vi "Boolean Array to Integer.vi"() -> ()   [LabVIEW 2010]
uses:
  <vilib>/DAQmx/write.llb/DAQmx Write (Digital 1D U8 1Chan NSamp).vi
panel:
  out "output array":u8[](array[numeric])
  out "unsigned 8bit integer":u8
  in  "Array":bool[](array[boolean])
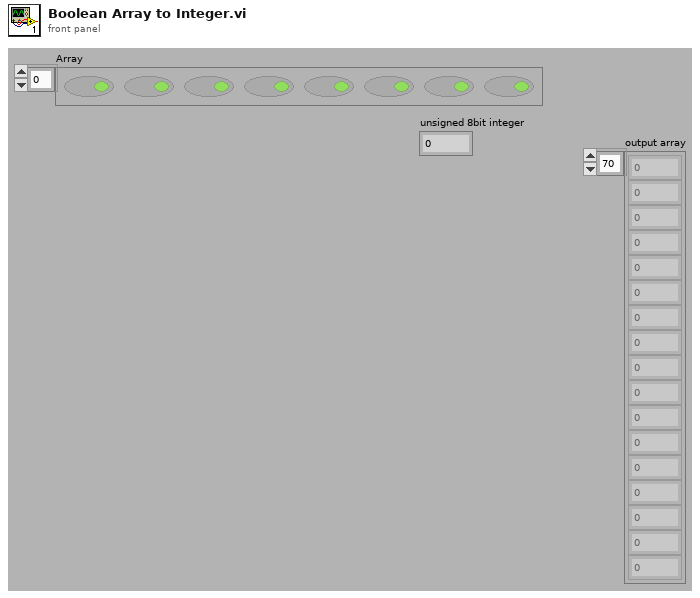
[diagram p1: front panel]
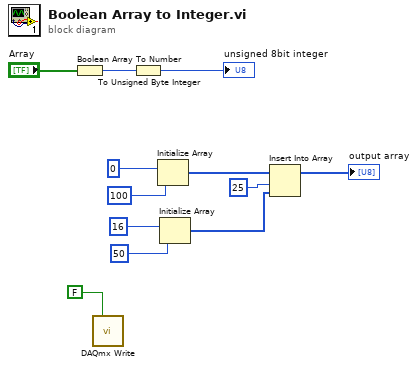
[diagram p0: block diagram]
diagram:
  n1 = Boolean Array To Number(Boolean array="Array") -> (number=w11:u32)
  n2 = call-poly <vilib>:"DAQmx Write.vi"("auto start"=FALSE) -> ()  [unwired: 12 in, 3 out]
  n3 = To Unsigned Byte Integer(number=w11) -> (unsigned 8bit integer=→"unsigned 8bit integer":u8)
  n4 = Initialize Array(u8 0 ("element"), 100 ("dimension size")) -> (w5:u8[])
  n5 = Initialize Array(u8 16 ("element"), 50 ("dimension size")) -> (w4:u8[])
  n6 = Insert Into Array(array=w5, index=25, new element=w4) -> (→"output array":u8[])
